vi "xcorr bkp delay.vi"(4 "shift":u8, 5 "Pulse Energy":fxp<+,32,0>=0.99609375, 6 "N":u8, 7 "y":u32, 8 "x":u32, 9 "enable":bool, 10 "lag":u16) -> (1 "Rxy valid":bool, 2 "Rxy":u64, 3 "trigger":bool)   [LabVIEW 2017]
uses:
  <vilib>/rvi/FXPMathLib/basic elements/FxpDiscreteDelay/XNode/nifxpmath_DiscreteDelay.xnode
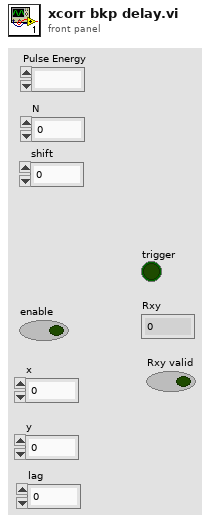
[diagram p1: front panel]
types:
  T1 = cluster{"Q":bool, "Q":bool, "Q":bool, "Q":bool, "Q":bool, "Q":bool, "Q":bool, "Q":bool, "Q":bool, "Q":bool, "Q":bool, "Q":bool, "Q":bool}
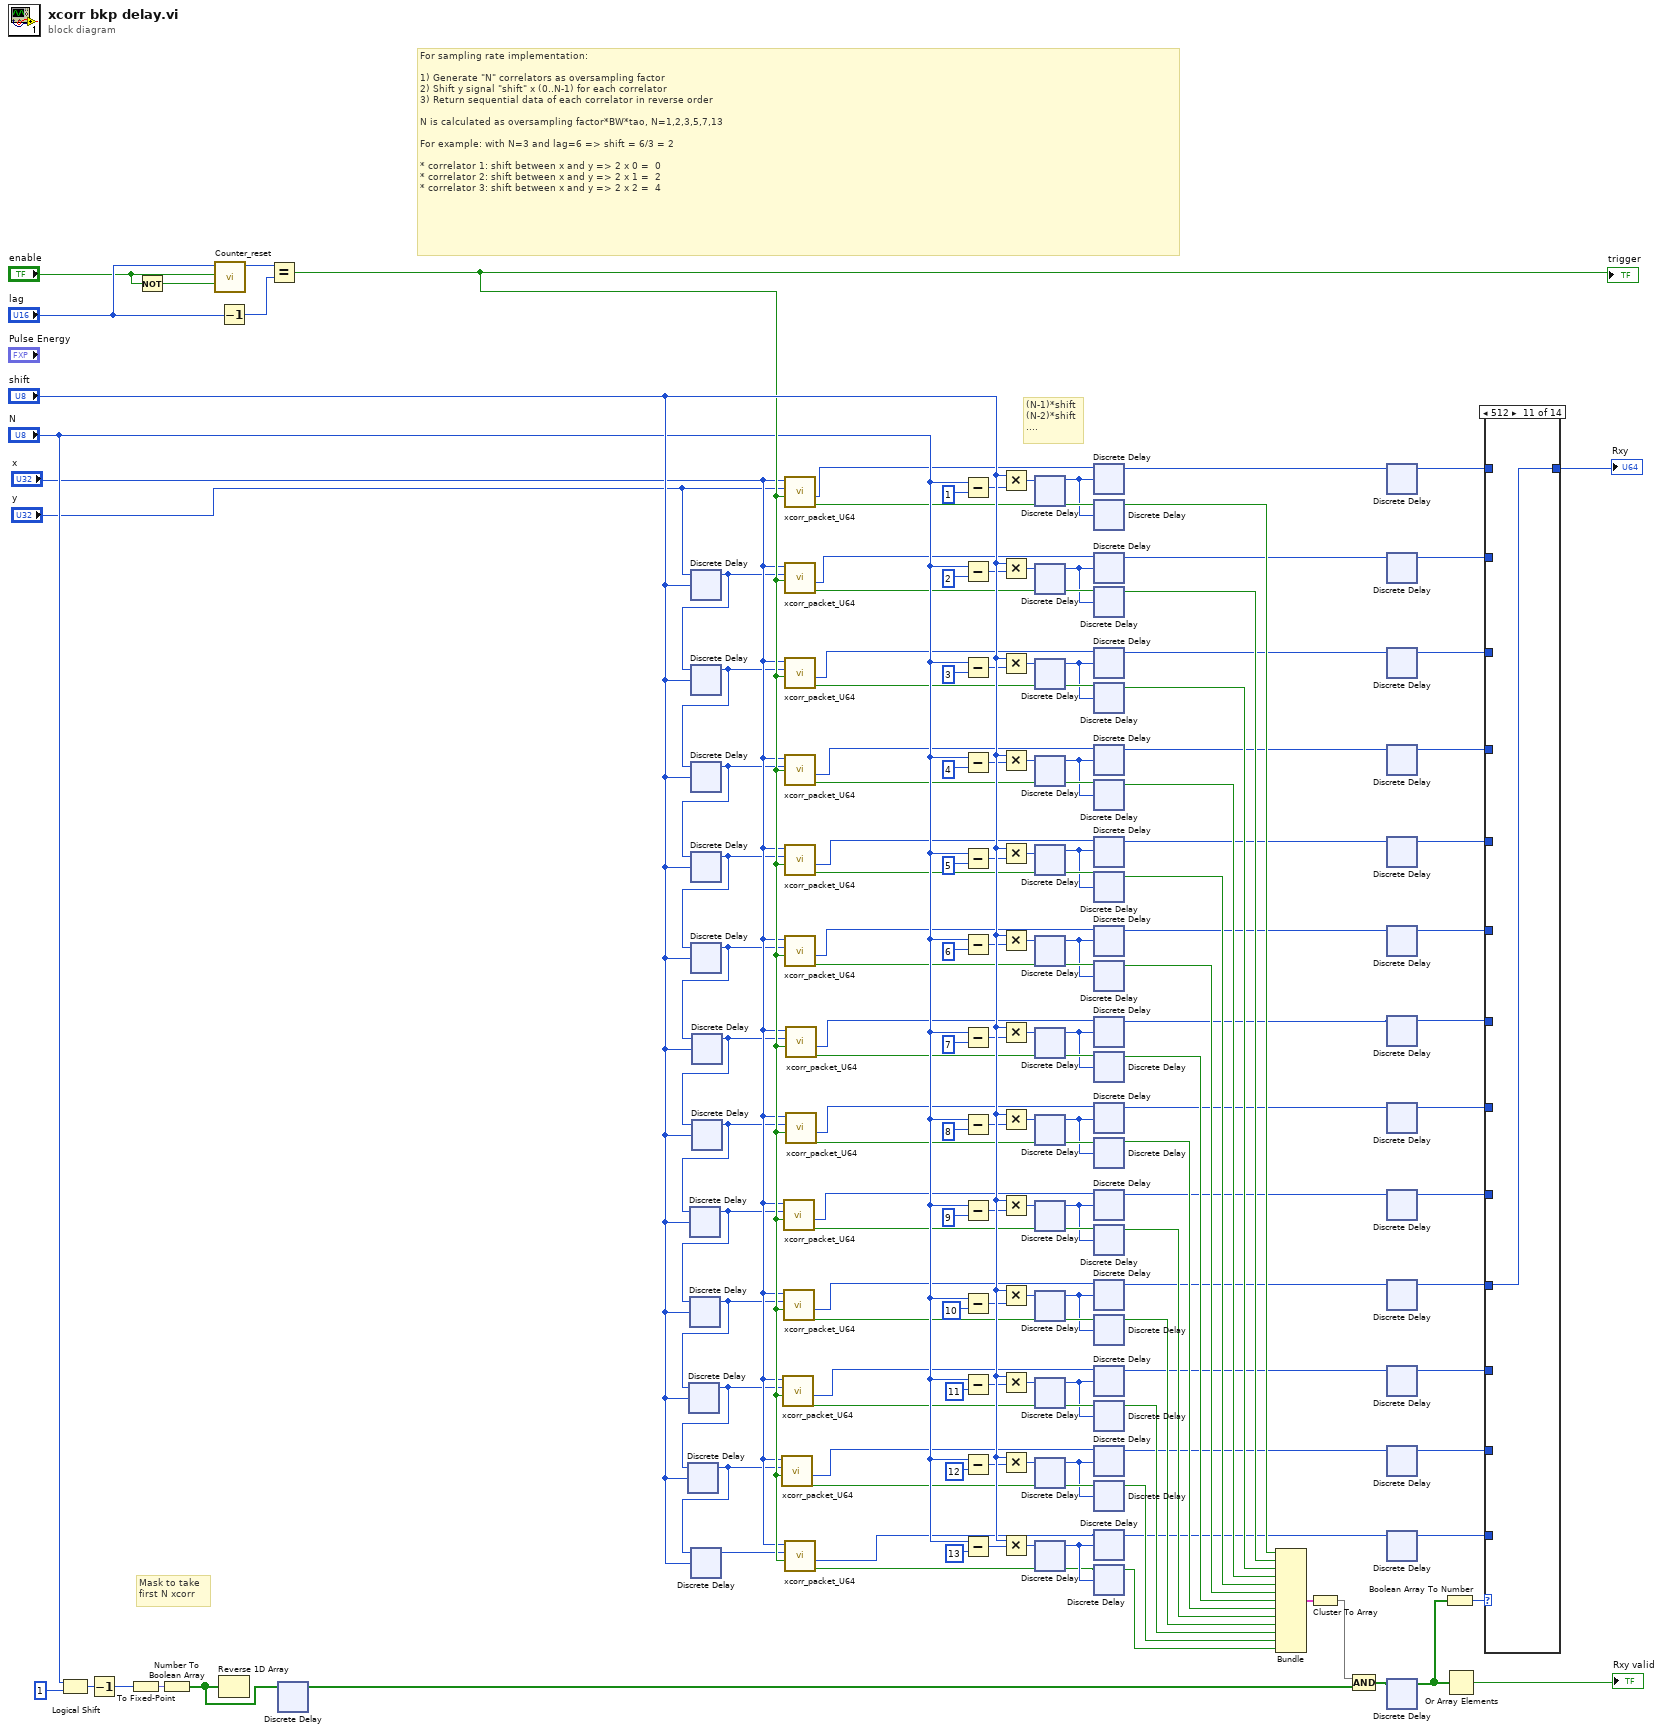
[diagram p0: block diagram]
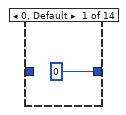
[diagram p2: hidden frame]
diagram:
  # "(N-1)*shift\n(N-2)*shift\n...."
  # "Mask to take \nfirst N xcorr"
  # "For sampling rate implementation:\n\n1) Generate \"N\" correlators as oversampling factor\n2) Shift y signal \"shift\" x (0..N-1) for each correlator\n3) Return sequential data of each correlator in reverse order\n\nN is calculated as oversampling factor*BW*tao, N=1,2,3,5,7,13\n\nFor example: with N=3 and lag=6 => shift = 6/3 = 2\n\n* correlator 1: shift between x and y => 2 x 0 =  0\n* correlator 2: shift between x and y => 2 x 1 =  2\n* correlator 3: shift between x and y => 2 x 2 =  4"
  n1 = Logical Shift(y="N", x=u16 1) -> (x << y=w144:u16)
  n2 = Decrement(x=w144) -> (x-1=w143:u16)
  n3 = To Fixed-Point(number=w143) -> (fixed-point=w142:fxp<+,13,13>)  [unwired: 1 in]
  n4 = Not(x="enable") -> (.not. x?=w151:bool)
  n5 = Number To Boolean Array(number=w142) -> (Boolean array=w140:bool[])
  n6 = call "Counter_reset.vi"("reset"=w151, "enable"="enable", "limit"="lag") -> ("count"=w152:u16)  [unwired: 8 in]
  n7 = Decrement(x="lag") -> (x-1=w149:u16)
  n8 = Reverse 1D Array(array=w140) -> ()  [unwired: 1 out]
  n9 = Equal?(x=w152, y=w149) -> (x = y?=w147:bool)
  "trigger" <- w147
  n10 = xnode ("Discrete Delay")("D"=w140) -> ("Q"=w32:bool[])
  n11 = xnode ("Discrete Delay")("D"="y", "n-1[0..255]"="shift") -> ("Q"=w90:u32)
  n12 = xnode ("Discrete Delay")("D"=w90, "n-1[0..255]"="shift") -> ("Q"=w100:u32)
  n13 = xnode ("Discrete Delay")("D"=w100, "n-1[0..255]"="shift") -> ("Q"=w99:u32)
  n14 = xnode ("Discrete Delay")("D"=w99, "n-1[0..255]"="shift") -> ("Q"=w98:u32)
  n15 = xnode ("Discrete Delay")("D"=w98, "n-1[0..255]"="shift") -> ("Q"=w97:u32)
  n16 = xnode ("Discrete Delay")("D"=w97, "n-1[0..255]"="shift") -> ("Q"=w96:u32)
  n17 = xnode ("Discrete Delay")("D"=w96, "n-1[0..255]"="shift") -> ("Q"=w95:u32)
  n18 = xnode ("Discrete Delay")("D"=w95, "n-1[0..255]"="shift") -> ("Q"=w94:u32)
  n19 = xnode ("Discrete Delay")("D"=w94, "n-1[0..255]"="shift") -> ("Q"=w93:u32)
  n20 = xnode ("Discrete Delay")("D"=w93, "n-1[0..255]"="shift") -> ("Q"=w92:u32)
  n21 = xnode ("Discrete Delay")("D"=w92, "n-1[0..255]"="shift") -> ("Q"=w91:u32)
  n22 = xnode ("Discrete Delay")("D"=w91, "n-1[0..255]"="shift") -> ("Q"=w122:u32)
  n23 = call "xcorr_packet_U64.vi"("x"="x", "y"=w91, "trigger"=w147) -> ("out"=w101:u64, "valid"=w105:bool)  [unwired: 5 in]
  n24 = call "xcorr_packet_U64.vi"("x"="x", "y"=w92, "trigger"=w147) -> ("out"=w102:u64, "valid"=w110:bool)  [unwired: 5 in]
  n25 = call "xcorr_packet_U64.vi"("x"="x", "y"=w94, "trigger"=w147) -> ("out"=w113:u64, "valid"=w112:bool)  [unwired: 5 in]
  n26 = call "xcorr_packet_U64.vi"("x"="x", "y"=w93, "trigger"=w147) -> ("out"=w103:u64, "valid"=w111:bool)  [unwired: 5 in]
  n27 = call "xcorr_packet_U64.vi"("x"="x", "y"="y", "trigger"=w147) -> ("out"=w137:u64, "valid"=w136:bool)  [unwired: 5 in]
  n28 = call "xcorr_packet_U64.vi"("x"="x", "y"=w90, "trigger"=w147) -> ("out"=w128:u64, "valid"=w133:bool)  [unwired: 5 in]
  n29 = call "xcorr_packet_U64.vi"("x"="x", "y"=w100, "trigger"=w147) -> ("out"=w127:u64, "valid"=w132:bool)  [unwired: 5 in]
  n30 = call "xcorr_packet_U64.vi"("x"="x", "y"=w99, "trigger"=w147) -> ("out"=w126:u64, "valid"=w130:bool)  [unwired: 5 in]
  n31 = call "xcorr_packet_U64.vi"("x"="x", "y"=w98, "trigger"=w147) -> ("out"=w123:u64, "valid"=w121:bool)  [unwired: 5 in]
  n32 = call "xcorr_packet_U64.vi"("x"="x", "y"=w97, "trigger"=w147) -> ("out"=w124:u64, "valid"=w125:bool)  [unwired: 5 in]
  n33 = call "xcorr_packet_U64.vi"("x"="x", "y"=w122, "trigger"=w147) -> ("out"=w38:u64, "valid"=w37:bool)  [unwired: 5 in]
  n34 = call "xcorr_packet_U64.vi"("x"="x", "y"=w96, "trigger"=w147) -> ("out"=w119:u64, "valid"=w118:bool)  [unwired: 5 in]
  n35 = call "xcorr_packet_U64.vi"("x"="x", "y"=w95, "trigger"=w147) -> ("out"=w114:u64, "valid"=w115:bool)  [unwired: 5 in]
  n36 = Subtract(x="N", y=u8 1 ("x")) -> (x-y=w87:u8)
  n37 = Subtract(x="N", y=u8 2 ("x")) -> (x-y=w85:u8)
  n38 = Subtract(x="N", y=u8 3 ("x")) -> (x-y=w83:u8)
  n39 = Subtract(x="N", y=u8 4 ("x")) -> (x-y=w81:u8)
  n40 = Subtract(x="N", y=u8 5 ("x")) -> (x-y=w79:u8)
  n41 = Subtract(x="N", y=u8 6 ("x")) -> (x-y=w77:u8)
  n42 = Subtract(x="N", y=u8 7 ("x")) -> (x-y=w75:u8)
  n43 = Subtract(x="N", y=u8 8 ("x")) -> (x-y=w73:u8)
  n44 = Subtract(x="N", y=u8 9 ("x")) -> (x-y=w71:u8)
  n45 = Subtract(x="N", y=u8 10 ("x")) -> (x-y=w69:u8)
  n46 = Subtract(x="N", y=u8 11 ("x")) -> (x-y=w67:u8)
  n47 = Subtract(x="N", y=u8 12 ("x")) -> (x-y=w66:u8)
  n48 = Subtract(x="N", y=u8 13 ("x")) -> (x-y=w63:u8)
  n49 = Multiply(x="shift", y=w87) -> (x*y=w65:u8)
  n50 = Multiply(x="shift", y=w85) -> (x*y=w62:u8)
  n51 = Multiply(x="shift", y=w83) -> (x*y=w60:u8)
  n52 = Multiply(x="shift", y=w81) -> (x*y=w58:u8)
  n53 = Multiply(x="shift", y=w79) -> (x*y=w56:u8)
  n54 = Multiply(x="shift", y=w77) -> (x*y=w54:u8)
  n55 = Multiply(x="shift", y=w75) -> (x*y=w52:u8)
  n56 = Multiply(x="shift", y=w73) -> (x*y=w50:u8)
  n57 = Multiply(x="shift", y=w71) -> (x*y=w48:u8)
  n58 = Multiply(x="shift", y=w69) -> (x*y=w46:u8)
  n59 = Multiply(x="shift", y=w67) -> (x*y=w44:u8)
  n60 = Multiply(x="shift", y=w66) -> (x*y=w42:u8)
  n61 = Multiply(x="shift", y=w63) -> (x*y=w40:u8)
  n62 = xnode ("Discrete Delay")("D"=w65) -> ("Q"=w64:u8)
  n63 = xnode ("Discrete Delay")("D"=w62) -> ("Q"=w61:u8)
  n64 = xnode ("Discrete Delay")("D"=w60) -> ("Q"=w59:u8)
  n65 = xnode ("Discrete Delay")("D"=w58) -> ("Q"=w57:u8)
  n66 = xnode ("Discrete Delay")("D"=w56) -> ("Q"=w55:u8)
  n67 = xnode ("Discrete Delay")("D"=w54) -> ("Q"=w53:u8)
  n68 = xnode ("Discrete Delay")("D"=w52) -> ("Q"=w51:u8)
  n69 = xnode ("Discrete Delay")("D"=w50) -> ("Q"=w49:u8)
  n70 = xnode ("Discrete Delay")("D"=w48) -> ("Q"=w47:u8)
  n71 = xnode ("Discrete Delay")("D"=w46) -> ("Q"=w45:u8)
  n72 = xnode ("Discrete Delay")("D"=w44) -> ("Q"=w43:u8)
  n73 = xnode ("Discrete Delay")("D"=w42) -> ("Q"=w41:u8)
  n74 = xnode ("Discrete Delay")("D"=w40) -> ("Q"=w39:u8)
  n75 = xnode ("Discrete Delay")("D"=w137, "n-1[0..255]"=w64) -> ("Q"=w26:u64)
  n76 = xnode ("Discrete Delay")("D"=w136, "n-1[0..255]"=w64) -> ("Q"=w135:bool)
  n77 = xnode ("Discrete Delay")("D"=w128, "n-1[0..255]"=w61) -> ("Q"=w24:u64)
  n78 = xnode ("Discrete Delay")("D"=w133, "n-1[0..255]"=w61) -> ("Q"=w134:bool)
  n79 = xnode ("Discrete Delay")("D"=w127, "n-1[0..255]"=w59) -> ("Q"=w22:u64)
  n80 = xnode ("Discrete Delay")("D"=w132, "n-1[0..255]"=w59) -> ("Q"=w131:bool)
  n81 = xnode ("Discrete Delay")("D"=w126, "n-1[0..255]"=w57) -> ("Q"=w20:u64)
  n82 = xnode ("Discrete Delay")("D"=w130, "n-1[0..255]"=w57) -> ("Q"=w129:bool)
  n83 = xnode ("Discrete Delay")("D"=w123, "n-1[0..255]"=w55) -> ("Q"=w18:u64)
  n84 = xnode ("Discrete Delay")("D"=w121, "n-1[0..255]"=w55) -> ("Q"=w120:bool)
  n85 = xnode ("Discrete Delay")("D"=w124, "n-1[0..255]"=w53) -> ("Q"=w16:u64)
  n86 = xnode ("Discrete Delay")("D"=w125, "n-1[0..255]"=w53) -> ("Q"=w34:bool)
  n87 = xnode ("Discrete Delay")("D"=w119, "n-1[0..255]"=w51) -> ("Q"=w14:u64)
  n88 = xnode ("Discrete Delay")("D"=w118, "n-1[0..255]"=w51) -> ("Q"=w117:bool)
  n89 = xnode ("Discrete Delay")("D"=w114, "n-1[0..255]"=w49) -> ("Q"=w12:u64)
  n90 = xnode ("Discrete Delay")("D"=w115, "n-1[0..255]"=w49) -> ("Q"=w109:bool)
  n91 = xnode ("Discrete Delay")("D"=w113, "n-1[0..255]"=w47) -> ("Q"=w10:u64)
  n92 = xnode ("Discrete Delay")("D"=w112, "n-1[0..255]"=w47) -> ("Q"=w108:bool)
  n93 = xnode ("Discrete Delay")("D"=w103, "n-1[0..255]"=w45) -> ("Q"=w8:u64)
  n94 = xnode ("Discrete Delay")("D"=w111, "n-1[0..255]"=w45) -> ("Q"=w107:bool)
  n95 = xnode ("Discrete Delay")("D"=w102, "n-1[0..255]"=w43) -> ("Q"=w6:u64)
  n96 = xnode ("Discrete Delay")("D"=w110, "n-1[0..255]"=w43) -> ("Q"=w106:bool)
  n97 = xnode ("Discrete Delay")("D"=w101, "n-1[0..255]"=w41) -> ("Q"=w4:u64)
  n98 = xnode ("Discrete Delay")("D"=w105, "n-1[0..255]"=w41) -> ("Q"=w104:bool)
  n99 = xnode ("Discrete Delay")("D"=w38, "n-1[0..255]"=w39) -> ("Q"=w2:u64)
  n100 = xnode ("Discrete Delay")("D"=w37, "n-1[0..255]"=w39) -> ("Q"=w36:bool)
  n101 = Bundle("Q"=w135, "Q"=w134, "Q"=w131, "Q"=w129, "Q"=w120, "Q"=w34, "Q"=w117, "Q"=w109, "Q"=w108, "Q"=w107, "Q"=w106, "Q"=w104, "Q"=w36) -> (w116:T1)  [unwired: 1 in]
  n102 = Cluster To Array(cluster=w116) -> (array=w89:bool[])
  n103 = Compound Arithmetic op=AND(w89, w32) -> (w30:bool[])
  n104 = xnode ("Discrete Delay")("D"=w26) -> ("Q"=w25:u64)
  n105 = xnode ("Discrete Delay")("D"=w24) -> ("Q"=w23:u64)
  n106 = xnode ("Discrete Delay")("D"=w22) -> ("Q"=w21:u64)
  n107 = xnode ("Discrete Delay")("D"=w20) -> ("Q"=w19:u64)
  n108 = xnode ("Discrete Delay")("D"=w18) -> ("Q"=w17:u64)
  n109 = xnode ("Discrete Delay")("D"=w16) -> ("Q"=w15:u64)
  n110 = xnode ("Discrete Delay")("D"=w14) -> ("Q"=w13:u64)
  n111 = xnode ("Discrete Delay")("D"=w12) -> ("Q"=w11:u64)
  n112 = xnode ("Discrete Delay")("D"=w10) -> ("Q"=w9:u64)
  n113 = xnode ("Discrete Delay")("D"=w8) -> ("Q"=w7:u64)
  n114 = xnode ("Discrete Delay")("D"=w6) -> ("Q"=w5:u64)
  n115 = xnode ("Discrete Delay")("D"=w4) -> ("Q"=w3:u64)
  n116 = xnode ("Discrete Delay")("D"=w2) -> ("Q"=w1:u64)
  n117 = xnode ("Discrete Delay")("D"=w30) -> ("Q"=w29:bool[])
  n118 = Boolean Array To Number(Boolean array=w29) -> (number=w35:u16)
  n119 = Or Array Elements(Boolean array=w29) -> (logical OR=→"Rxy valid":bool)
  n120 = case shown="512" w35 {
    tunnel: [u64 0 ("out") w154 w155 w156 w157 w158 w159 w160 w161 w162 w163 w164 w165 w166] -> w27
    tunnel: w25 -> [_ w154 _ _ _ _ _ _ _ _ _ _ _ _]
    tunnel: w23 -> [_ _ w155 _ _ _ _ _ _ _ _ _ _ _]
    tunnel: w21 -> [_ _ _ w156 _ _ _ _ _ _ _ _ _ _]
    tunnel: w19 -> [_ _ _ _ w157 _ _ _ _ _ _ _ _ _]
    tunnel: w17 -> [_ _ _ _ _ w158 _ _ _ _ _ _ _ _]
    tunnel: w15 -> [_ _ _ _ _ _ w159 _ _ _ _ _ _ _]
    tunnel: w1 -> [_ _ _ _ _ _ _ _ _ _ _ _ _ w166]
    tunnel: w13 -> [_ _ _ _ _ _ _ w160 _ _ _ _ _ _]
    tunnel: w11 -> [_ _ _ _ _ _ _ _ w161 _ _ _ _ _]
    tunnel: w9 -> [_ _ _ _ _ _ _ _ _ w162 _ _ _ _]
    tunnel: w5 -> [_ _ _ _ _ _ _ _ _ _ _ w164 _ _]
    tunnel: w3 -> [_ _ _ _ _ _ _ _ _ _ _ _ w165 _]
    tunnel: w7 -> [_ _ _ _ _ _ _ _ _ _ w163 _ _ _]
    frame 0, Default {
    }
    frame 1 {
    }
    frame 2 {
    }
    frame 4 {
    }
    frame 8 {
    }
    frame 16 {
    }
    frame 32 {
    }
    frame 64 {
    }
    frame 128 {
    }
    frame 256 {
    }
    frame 512 {
    }
    frame 1024 {
    }
    frame 2048 {
    }
    frame 4096 {
    }
  }
  "Rxy" <- w27
